vi "MAIN_UI.vi"() -> ()   [LabVIEW 2019]
uses:
  SV_Wrap/shared variable info.ctl
  SV_Wrap/SharedVariableWrapper.lvclass
  Logger_class/Current Alarms.ctl
  Logger_class/EventData.ctl
  TypeDef/AlarmType.ctl
  SV_Wrap/SharedVariableWrapper.lvclass/SharedVariableWrapper.ctl
  TypeDef/error.ctl
  GUI_class/GUI.lvclass/GUI.ctl
  MessageAMC_class/MessageAMC.lvclass
  C:/Users/ANENKOV_V1/Desktop/SRC_H400/src/MessageInterface_class/MessageInterface.lvclass
  ConfigJSON_class/ConfigJSON.lvclass
  TypeDef/Windows.ctl
  GUI Sensor Lib/GUI Sensor Lib.lvclass
  C:/Users/ANENKOV_V1/Desktop/SRC_H400/src/GUI_class/GUI.lvclass
  GUI Alarm Setting/GUI Alarm Setting.lvclass
  GUI Data Viewer_class/GUI Data Viewer.lvclass
  GUI Test Channels_class/GUI Test Channels.lvclass
  GUI Setting_class/GUI Setting.lvclass
  GUI Test HIPRESS_class/GUI Test HIPRESS.lvclass
  GUI NV class/GUI NV.lvclass
  GUI Work Windows_class/GUI Work Windows.lvclass
  PumpMotorGroup_class/GUI PumpMotorGroup.lvclass
  ConfigJSON_class/ConfigJSON.lvclass/ConfigJSON.ctl
  28b6755c-365d-47ee-a391-b63f47e4b467.vi
  4313fddc-c2f7-4c5c-84fc-ac29d5ff3ebf.vi
  d1d2263f-3a8b-4136-8dd0-7d9082776734.vi
  28b6755c-365d-47ee-a391-b63f47e4b467.vi/59a5e995-9048-4616-a220-4159bcf9e391.vi
  SV_Wrap/Write Var Info.vi
  SV_Wrap/Read Var Info.vi
  4313fddc-c2f7-4c5c-84fc-ac29d5ff3ebf.vi/c3b15906-7c69-4354-9ca0-0932e3ff86b4.vi
  GUI_class/Set Win State.vi
  GUI_class/protected/GetSheredData.vi
  SV_Wrap/Read connection str.vi
  <userlib>/_OpenG.lib/time/time.llb/Tick Count (ms)__ogtk.vi
  <vilib>/Platform/browser.llb/Open URL in Default Browser (string).vi
  GUI_class/GUI.lvclass
  <vilib>/NI/AMC/AMC.lvlib
  MessageInterface_class/MessageInterface.lvclass
panel:
  in  "grafana":bool
  out "База данных":bool
  out "Контролер":bool
  in  "Clear error":bool
  in  "Boolean":bool
  out "SVW":refnum<class "SharedVariableWrapper.lvclass">
  in  "Log Out":bool
  in  "Log In":bool
  out "Multicolumn Listbox":i32(listbox)=-1
  out "map":map{string, T1}(c390)
  in  "GUI PMG":bool
  in  "NV2":bool
  in  "NV1":bool
  in  "HI press":bool
  in  "Channel Testing":bool
  in  "Data":bool
  in  "Start Button":bool
  in  "Settings Channels":bool
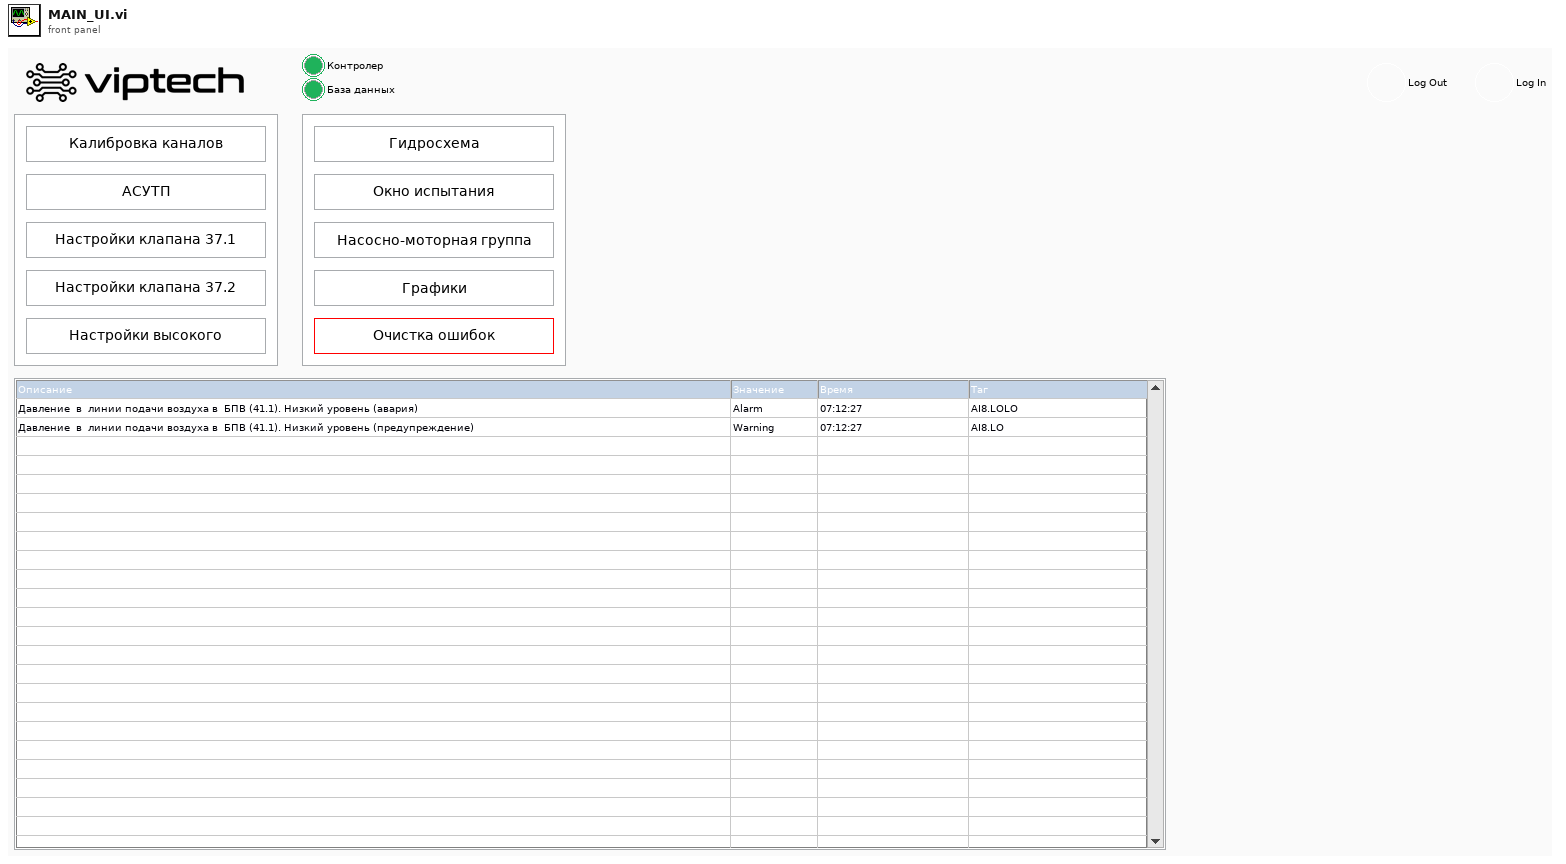
[diagram p1: front panel]
types:
  T1 = typedef "SharedVariableWrapper.lvclass/shared variable info.ctl" = cluster{"shared variable":refnum<k21>, "connected":bool, "Value":variant, "UpdateTime":timestamp}
  T2 = typedef "Current Alarms.ctl" = cluster{"alarms":T3[]}
  T3 = typedef "EventData.ctl" = cluster{"obj_tag":string, "event_tag":string, "Description":string, "ALARM TYPE":T4, "Value DBL":dbl, "Value INT":i32, "Value STR":string, "Time Stamp":timestamp}
  T4 = typedef "AlarmType.ctl" = enum16{"Normal", "Warning", "Alarm"}
  T5 = typedef "error.ctl" = errorcluster
  T6 = enum32{"Invalid", "Standard", "Closed", "Hidden", "Minimized", "Maximized"}
  T7 = enum32{"invalid app kind", "Development System", "Run Time System", "Student Edition", "Embedded LabVIEW", "Evaluation", "Custom"}
  T8 = typedef "Windows.ctl" = cluster{"GUI Sensor Lib":refnum<class "GUI Sensor Lib.lvclass">, "GUI Alarm Setting":refnum<class "GUI Alarm Setting.lvclass">, "GUI Data Viewer":refnum<class "GUI Data Viewer.lvclass">, "GUI Test Channels":refnum<class "GUI Test Channels.lvclass">, "GUI Setting":refnum<class "GUI Setting.lvclass">, "GUI Test HIPRESS":refnum<class "GUI Test HIPRESS.lvclass">, "GUI NV 1":refnum<class "GUI NV.lvclass">, "GUI NV 2":refnum<class "GUI NV.lvclass">, "GUI Work Windows":refnum<class "GUI Work Windows.lvclass">, "GUI PMG 2":refnum<class "GUI PumpMotorGroup.lvclass">}
  T9 = typedef "SharedVariableWrapper.lvclass/Config.ctl" = cluster{"connection str":string, "timeout":dbl, "ip":string}
  T10 = cluster{"Core":cluster{"Current VI Reference":refnum<vi>, "Close Panel on Exit?":bool}, "JSON":refnum<class "ConfigJSON.lvclass">, "SVW":refnum<class "SharedVariableWrapper.lvclass">, "amc":refnum<class "MessageAMC.lvclass">, "Windows":T8}
  T11 = cluster{"Current VI Reference":refnum<vi>, "Close Panel on Exit?":bool}
  T12 = typedef "GUI Paths.ctl" = cluster{"Dir Data":path, "Dir Setting":path, "SensorLib":path, "Dir Scripts":path}
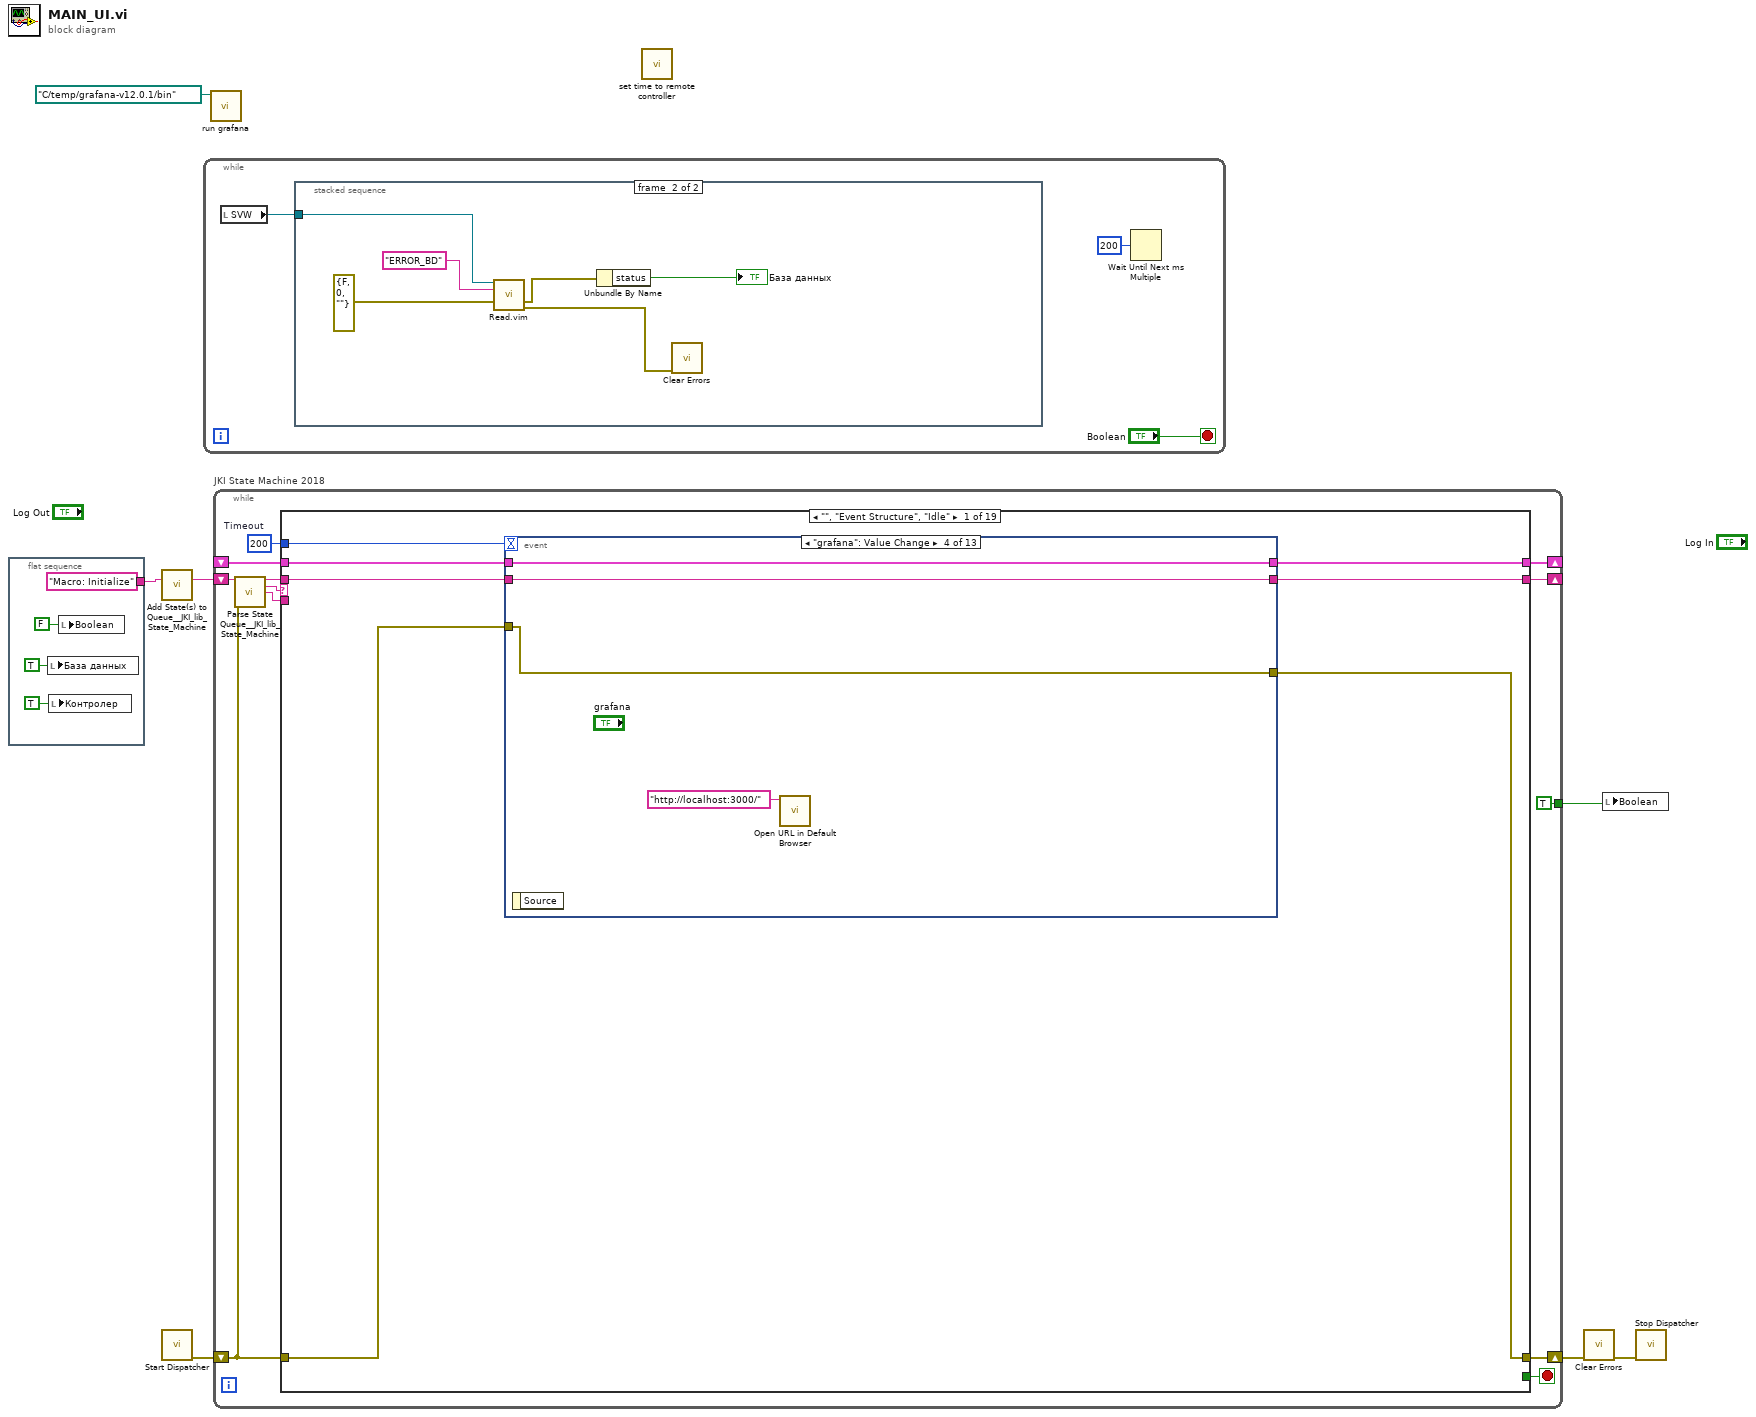
[diagram p0: block diagram]
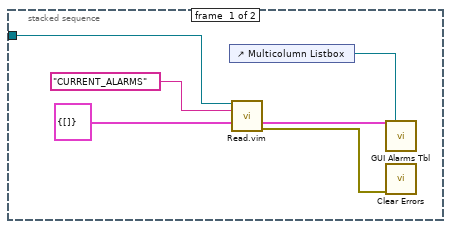
[diagram p2: hidden frame]
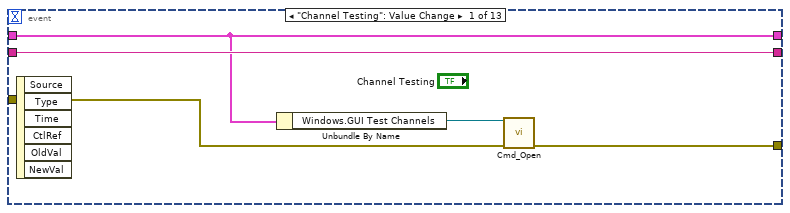
[diagram p3: hidden frame]
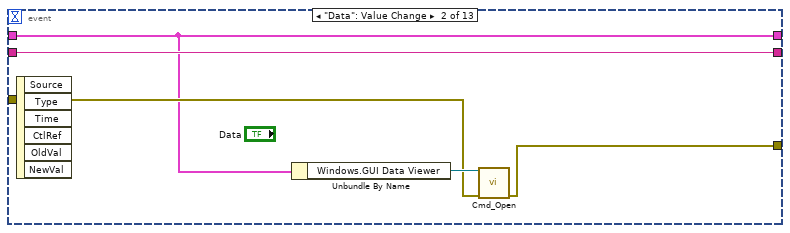
[diagram p4: hidden frame]
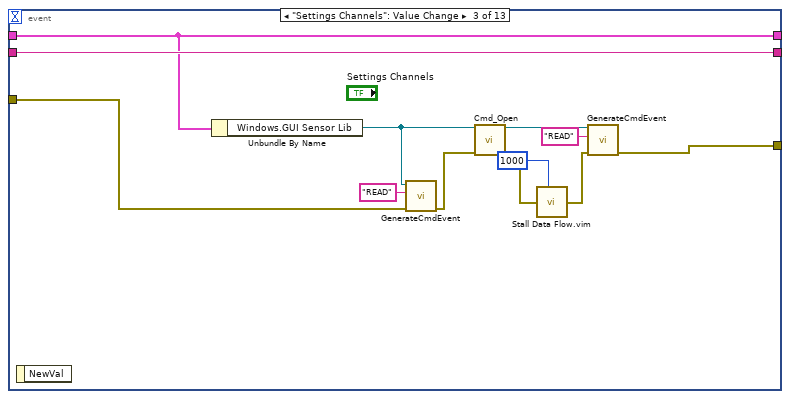
[diagram p5: hidden frame]
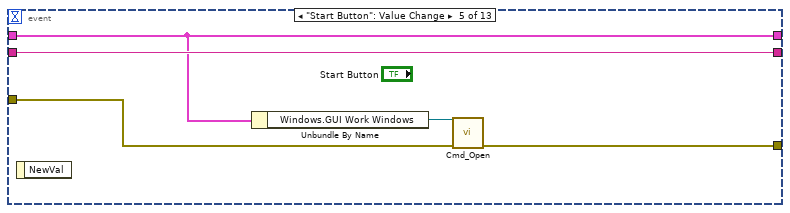
[diagram p6: hidden frame]
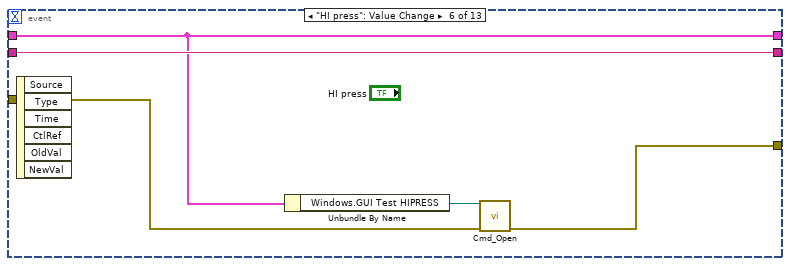
[diagram p7: hidden frame]
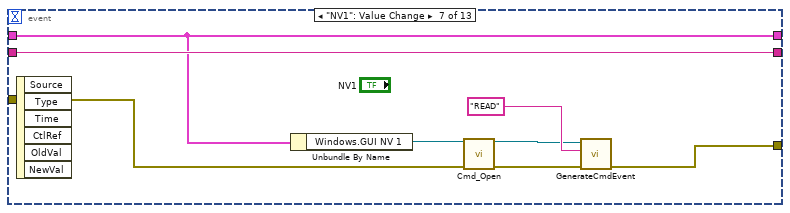
[diagram p8: hidden frame]
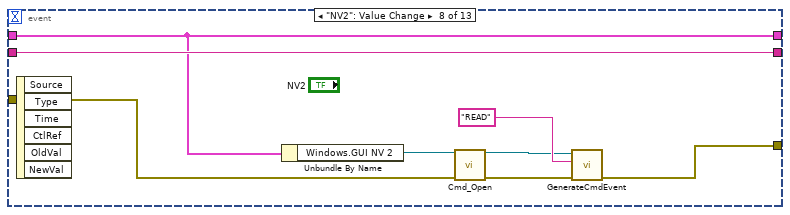
[diagram p9: hidden frame]
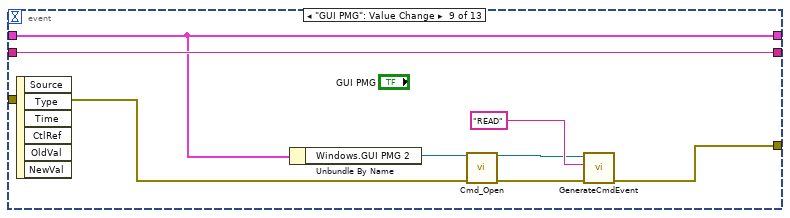
[diagram p10: hidden frame]
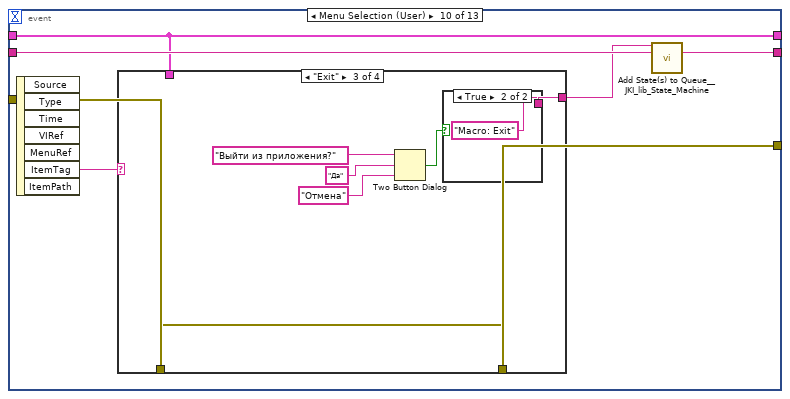
[diagram p11: hidden frame]
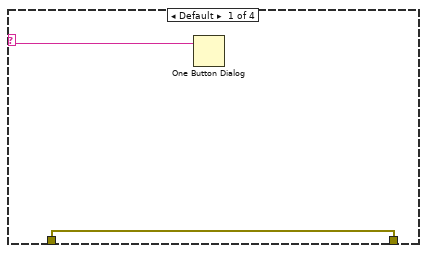
[diagram p12: hidden frame]
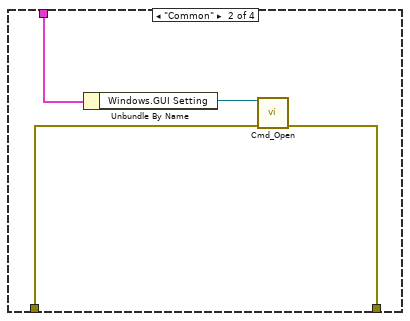
[diagram p13: hidden frame]
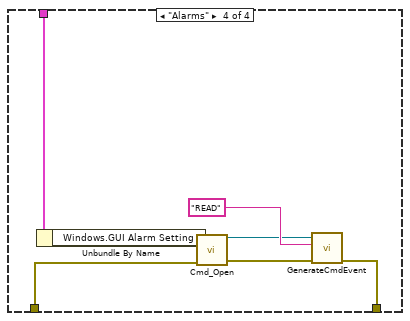
[diagram p15: hidden frame]
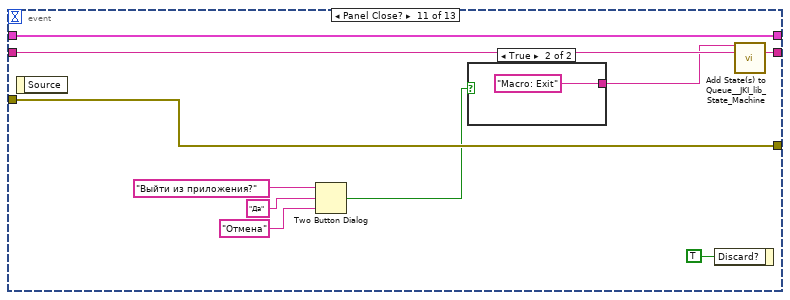
[diagram p16: hidden frame]
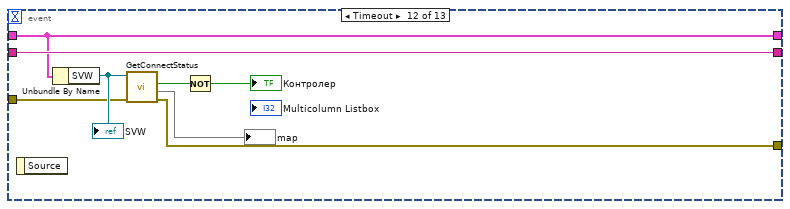
[diagram p18: hidden frame]
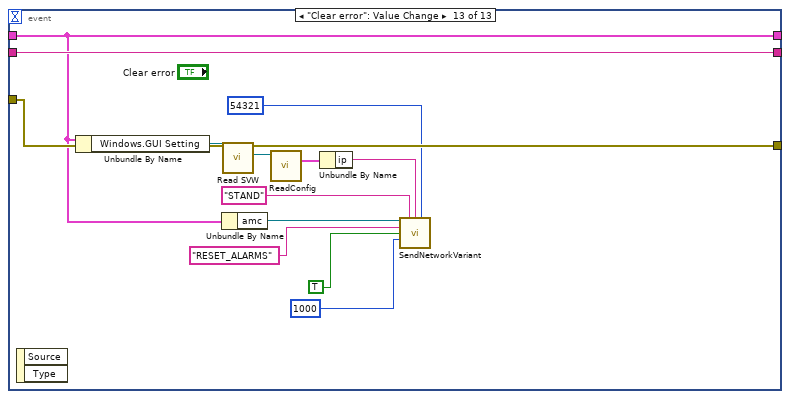
[diagram p19: hidden frame]
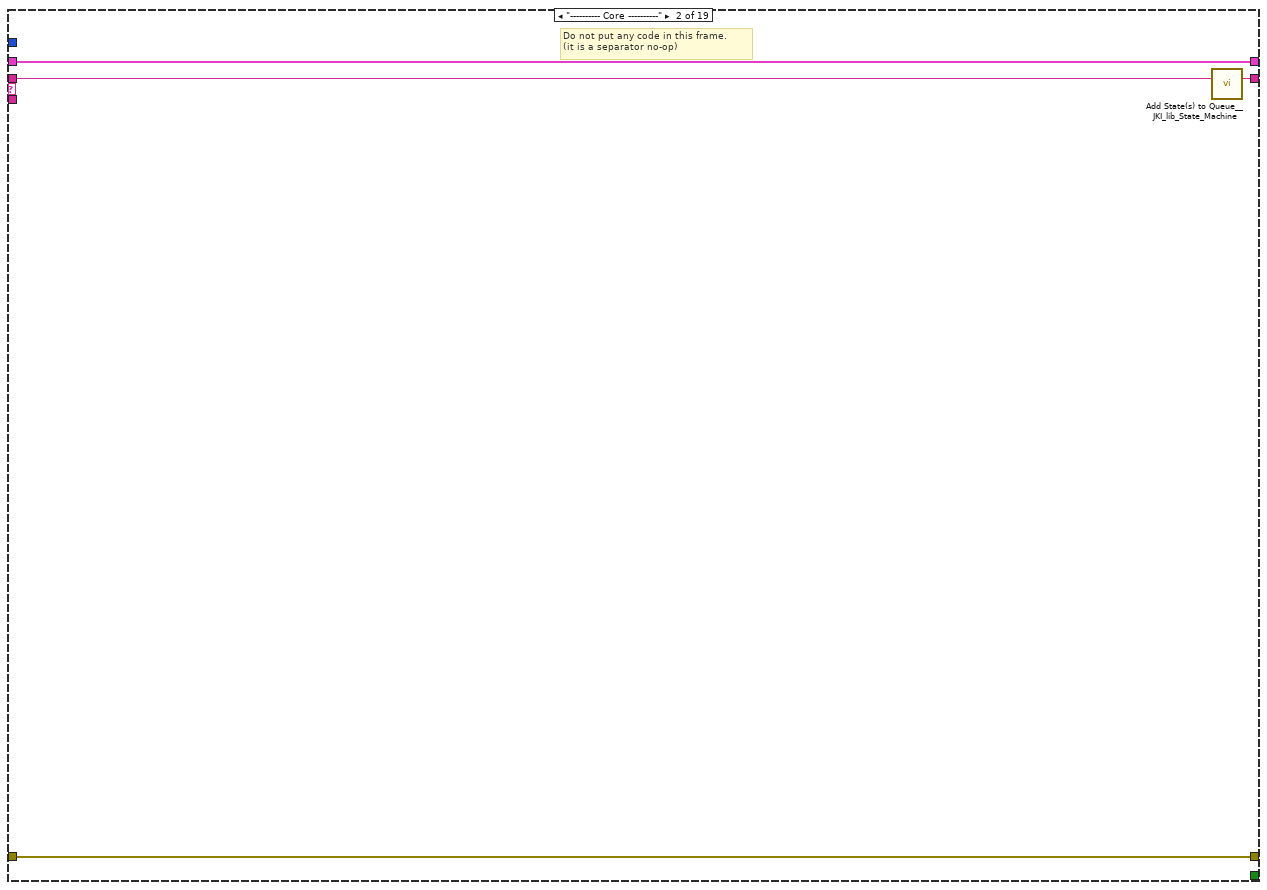
[diagram p20: hidden frame]
diagram:
  n1 = flat-sequence {
    tunnel: ["Macro: Initialize"] -> w2
    frame #0 {
      n2 = local write "База данных"(TRUE ("База данных")) -> ()
      n3 = local write "Контролер"(TRUE ("Контролер")) -> ()
      n4 = local write "Boolean"(FALSE ("Boolean")) -> ()
    }
  }
  n5 = call <vilib>:"Add State(s) to Queue__JKI_lib_State_Machine.vi"("State(s) in (\"\")"=w2) -> ("States Out"=w7:string)  [unwired: 14 in]
  n6 = call <vilib>:"Start Dispatcher.vi"() -> ("error out"=w6:errorcluster)  [unwired: 13 in, 2 out]
  n7 = while {
    stop <- "Boolean" stop-if-true
    n8 = local read "SVW"() -> (w14:refnum<class "SharedVariableWrapper.lvclass">)
    n9 = stacked-sequence {
      tunnel: w14 -> [w16 w25]
      frame #0 {
        n10 = control-ref of="Multicolumn Listbox"() -> (w20:refnum<vi>)
        n11 = call "Read.vim"("SharedVariableWrapper in"=w16, "name"="CURRENT_ALARMS", "DataType"=T2 {"alarms"=[]} ("data out")) -> ("data out"=w19:T2, "error out"=w18:errorcluster)  [unwired: 6 in, 5 out]
        n12 = call "GUI Alarms Tbl.vi"("data in"=w19, "Multicolumn Listbox ref"=w20) -> ()  [unwired: 12 in, 2 out]
        n13 = call <vilib>:"Clear Errors.vi"("error in (no error)"=w18) -> ()  [unwired: 5 in, 2 out]
      }
      frame #1 {
        n14 = call "Read.vim"("SharedVariableWrapper in"=w25, "name"="ERROR_BD", "DataType"=T5 {"status"=FALSE, "code"=0, "source"=""} ("error")) -> ("data out"=w22:T5, "error out"=w24:errorcluster)  [unwired: 6 in, 5 out]
        n15 = Unbundle By Name(w22) -> ("status"=→"База данных":bool)
        n16 = call <vilib>:"Clear Errors.vi"("error in (no error)"=w24) -> ()  [unwired: 5 in, 2 out]
      }
    }
    n17 = Wait Until Next ms Multiple(millisecond multiple=u32 200) -> ()  [unwired: 1 out]
  }
  n18 = call "run grafana.vi"("working directory"=path "C:/temp/grafana-v12.0.1/bin") -> ()  [unwired: 11 in]
  n19 = while "JKI State Machine 2018" {
    shift-right: [w31] -> _
    shift-left: _ -> [w30]
    shift-right: [w34] -> w5
    shift-left: w6 -> [w28]
    shift-right: [w33] -> _
    shift-left: w7 -> [w35]
    tunnel: [TRUE ("Boolean")] -> w3
    stop <- w32 stop-if-true
    w29 = 200  # Timeout
    n20 = call <vilib>:"Parse State Queue__JKI_lib_State_Machine.vi"("State Queue"=w35, "Error In (no error)"=w28) -> ("Remaining States"=w37:string, "Current State"=w38:string, "Arguments"=w36:string)  [unwired: 11 in]
    n21 = case shown="\"\", \"Event Structure\", \"Idle\"" w38 {
      selector: w38 -> [_ _ w169 _ _ _ _ _ _ _ _ _ _ _ _ _ _ _ _]
      tunnel: w37 -> [w45 w168 w173 w192 w198 w203 w207 w225 w231 w235 w239 w245 w256 w325 w330 w341 w345 w350 w361]
      tunnel: w36 -> [_ _ _ _ _ _ _ _ _ _ _ w240 w250 _ _ _ _ _ _]
      tunnel: w30 -> [w43 w165 w171 w185 w195 w201 w204 _ w226 w232 w237 w243 w252 w322 w327 w338 w342 w348 w358]
      tunnel: [w42 w166 w175 w189 errorcluster {"status"=FALSE, "code"=0, "source"=""} ("error out") w200 w205 w210 w227 w233 w236 w241 w253 w323 w328 w339 w343 w349 w359] -> w34
      tunnel: w28 -> [w41 w166 w174 w189 w194 w200 w205 w220 w228 w233 w236 w242 w254 w323 w328 w339 w343 w347 w360]
      tunnel: [w44 w167 w172 w191 w197 w202 w206 w225 w230 w234 w238 w244 w255 w324 w329 w340 w344 w350 w361] -> w33
      tunnel: [_ _ _ _ _ TRUE _ _ _ _ _ _ _ _ _ _ _ _ _] -> w32
      tunnel: [w40 w165 w171 w190 w195 w201 w204 w224 w226 w232 w237 w243 w252 w322 w327 w338 w342 w346 w358] -> w31
      tunnel: w29 -> [w39 _ _ _ _ _ _ _ _ _ _ _ _ _ _ _ _ _ _]
      frame "", "Event Structure", "Idle" {
        n22 = event shown="[3] \"grafana\": Value Change" {
          selector: _ -> [_ _ _ _ _ _ _ _ _ _ _ _ _]
          dyn-events: _ -> [_ _ _ _ _ _ _ _ _ _ _ _ _]
          timeout: w39 -> [_ _ _ _ _ _ _ _ _ _ _ _ _]
          tunnel: w45 -> [w50 w55 w67 w71 w76 w81 w89 w97 w105 w110 w142 w151 w164]
          tunnel: [w50 w55 w67 w71 w76 w81 w89 w97 w105 w111 w141 w151 w164] -> w44
          tunnel: w43 -> [w47 w51 w66 w69 w75 w79 w87 w95 w103 w108 w139 w150 w153]
          tunnel: [w46 w52 w65 w70 w73 w77 w85 w93 w101 w106 w140 w149 w163] -> w42
          tunnel: w41 -> [w48 w53 w60 w70 w74 w78 w86 w94 w102 w107 w140 w147 w163]
          tunnel: [w47 w51 w66 w69 w75 w79 w87 w95 w103 w108 w139 w150 w153] -> w40
          event "Channel Testing": Value Change {
            n23 = event-data() -> ()  [unwired: 1 in, 6 out]
            n24 = Unbundle By Name(w47) -> ("Windows.GUI Test Channels"=w49:refnum<class "GUI Test Channels.lvclass">)
            n25 = call "Cmd_Open.vi"("reference in"=w49, "error in (no error)"=w48) -> ("error out"=w46:errorcluster)  [unwired: 12 in, 1 out]
          }
          event "Data": Value Change {
            n26 = event-data() -> ()  [unwired: 1 in, 6 out]
            n27 = Unbundle By Name(w51) -> ("Windows.GUI Data Viewer"=w54:refnum<class "GUI Data Viewer.lvclass">)
            n28 = call "Cmd_Open.vi"("reference in"=w54, "error in (no error)"=w53) -> ("error out"=w52:errorcluster)  [unwired: 12 in, 1 out]
          }
          event "Settings Channels": Value Change {
            n29 = event-data() -> ()  [unwired: 1 in, 1 out]
            n30 = Unbundle By Name(w66) -> ("Windows.GUI Sensor Lib"=w61:refnum<class "GUI Sensor Lib.lvclass">)
            n31 = call "GenerateCmdEvent.vi"("error in (no error)"=w60, "CMD"="READ", "GUI in"=w61) -> ("error out"=w59:errorcluster)  [unwired: 7 in, 1 out]
            n32 = call "Cmd_Open.vi"("reference in"=w61, "error in (no error)"=w59) -> ("reference out"=w64:refnum<class "GUI Sensor Lib.lvclass">, "error out"=w58:errorcluster)  [unwired: 12 in]
            n33 = call "Stall Data Flow.vim"("value in"=w58, "milliseconds to wait"=u32 1000) -> ("value out"=w57:errorcluster)  [unwired: 1 out]
            n34 = call "GenerateCmdEvent.vi"("error in (no error)"=w57, "CMD"="READ", "GUI in"=w64) -> ("error out"=w65:errorcluster)  [unwired: 7 in, 1 out]
          }
          event "grafana": Value Change {
            n35 = event-data() -> ()  [unwired: 1 in, 1 out]
            n36 = call-poly <vilib>:"Open URL in Default Browser.vi"("URL"="http://localhost:3000/") -> ()  [unwired: 5 in, 2 out]
          }
          event "Start Button": Value Change {
            n37 = event-data() -> ()  [unwired: 1 in, 1 out]
            n38 = Unbundle By Name(w75) -> ("Windows.GUI Work Windows"=w72:refnum<class "GUI Work Windows.lvclass">)
            n39 = call "Cmd_Open.vi"("reference in"=w72, "error in (no error)"=w74) -> ("error out"=w73:errorcluster)  [unwired: 12 in, 1 out]
          }
          event "HI press": Value Change {
            n40 = event-data() -> ()  [unwired: 1 in, 6 out]
            n41 = Unbundle By Name(w79) -> ("Windows.GUI Test HIPRESS"=w80:refnum<class "GUI Test HIPRESS.lvclass">)
            n42 = call "Cmd_Open.vi"("reference in"=w80, "error in (no error)"=w78) -> ("error out"=w77:errorcluster)  [unwired: 12 in, 1 out]
          }
          event "NV1": Value Change {
            n43 = event-data() -> ()  [unwired: 1 in, 6 out]
            n44 = Unbundle By Name(w87) -> ("Windows.GUI NV 1"=w88:refnum<class "GUI NV.lvclass">)
            n45 = call "Cmd_Open.vi"("reference in"=w88, "error in (no error)"=w86) -> ("reference out"=w82:refnum<class "GUI NV.lvclass">, "error out"=w83:errorcluster)  [unwired: 12 in]
            n46 = call "GenerateCmdEvent.vi"("error in (no error)"=w83, "CMD"="READ", "GUI in"=w82) -> ("error out"=w85:errorcluster)  [unwired: 7 in, 1 out]
          }
          event "NV2": Value Change {
            n47 = event-data() -> ()  [unwired: 1 in, 6 out]
            n48 = Unbundle By Name(w95) -> ("Windows.GUI NV 2"=w96:refnum<class "GUI NV.lvclass">)
            n49 = call "Cmd_Open.vi"("reference in"=w96, "error in (no error)"=w94) -> ("reference out"=w90:refnum<class "GUI NV.lvclass">, "error out"=w91:errorcluster)  [unwired: 12 in]
            n50 = call "GenerateCmdEvent.vi"("error in (no error)"=w91, "CMD"="READ", "GUI in"=w90) -> ("error out"=w93:errorcluster)  [unwired: 7 in, 1 out]
          }
          event "GUI PMG": Value Change {
            n51 = event-data() -> ()  [unwired: 1 in, 6 out]
            n52 = Unbundle By Name(w103) -> ("Windows.GUI PMG 2"=w104:refnum<class "GUI PumpMotorGroup.lvclass">)
            n53 = call "Cmd_Open.vi"("reference in"=w104, "error in (no error)"=w102) -> ("reference out"=w98:refnum<class "GUI PumpMotorGroup.lvclass">, "error out"=w99:errorcluster)  [unwired: 12 in]
            n54 = call "GenerateCmdEvent.vi"("error in (no error)"=w99, "CMD"="READ", "GUI in"=w98) -> ("error out"=w101:errorcluster)  [unwired: 7 in, 1 out]
          }
          event Menu Selection (User) {
            n55 = event-data() -> ("ItemTag"=w112:string)  [unwired: 1 in, 6 out]
            n56 = case shown="\"Exit\"" w112 {
              selector: w112 -> [w113 _ _ _]
              tunnel: [_ _ w124 _] -> w109
              tunnel: w108 -> [_ w117 _ w130]
              tunnel: w107 -> [w114 w116 w123 w131]
              tunnel: [w114 w115 w123 w126] -> w106
              frame Default {
                n57 = One Button Dialog(message=w113) -> ()  [unwired: 1 in, 1 out]
              }
              frame "Common" {
                n58 = Unbundle By Name(w117) -> ("Windows.GUI Setting"=w118:refnum<class "GUI Setting.lvclass">)
                n59 = call "Cmd_Open.vi"("reference in"=w118, "error in (no error)"=w116) -> ("error out"=w115:errorcluster)  [unwired: 12 in, 1 out]
              }
              frame "Exit" {
                n60 = Two Button Dialog(message="Выйти из приложения?", 1:"Отмена" ("F button name (\"Cancel\")"), 2:"Да" ("T button name (\"OK\")")) -> (T button?=w119:bool)
                n61 = case shown="True" w119 {
                  tunnel: [_ "Macro: Exit"] -> w124
                  frame False {
                  }
                  frame True {
                  }
                }
              }
              frame "Alarms" {
                n62 = Unbundle By Name(w130) -> ("Windows.GUI Alarm Setting"=w132:refnum<class "GUI Alarm Setting.lvclass">)
                n63 = call "Cmd_Open.vi"("reference in"=w132, "error in (no error)"=w131) -> ("reference out"=w128:refnum<class "GUI Alarm Setting.lvclass">, "error out"=w127:errorcluster)  [unwired: 12 in]
                n64 = call "GenerateCmdEvent.vi"("error in (no error)"=w127, "CMD"="READ", "GUI in"=w128) -> ("error out"=w126:errorcluster)  [unwired: 7 in, 1 out]
              }
            }
            n65 = call <vilib>:"Add State(s) to Queue__JKI_lib_State_Machine.vi"("State(s) in Front (\"\")"=w109, "State(s) in (\"\")"=w110) -> ("States Out"=w111:string)  [unwired: 13 in]
          }
          event Panel Close? {
            n66 = event-data() -> ()  [unwired: 1 in, 1 out]
            n67 = Two Button Dialog(message="Выйти из приложения?", 1:"Отмена" ("F button name (\"Cancel\")"), 2:"Да" ("T button name (\"OK\")")) -> (T button?=w133:bool)
            n68 = case shown="True" w133 {
              tunnel: [_ "Macro: Exit"] -> w138
              frame False {
              }
              frame True {
              }
            }
            n69 = event-data("Discard?"=TRUE) -> ()  [unwired: 1 in, 1 out]
            n70 = call <vilib>:"Add State(s) to Queue__JKI_lib_State_Machine.vi"("State(s) in Front (\"\")"=w138, "State(s) in (\"\")"=w142) -> ("States Out"=w141:string)  [unwired: 13 in]
          }
          event Timeout {
            n71 = event-data() -> ()  [unwired: 1 in, 1 out]
            n72 = Unbundle By Name(w150) -> ("SVW"=w148:refnum<class "SharedVariableWrapper.lvclass">)
            "SVW" <- w148
            n73 = call "GetConnectStatus.vi"("error in (no error)"=w147, "SharedVariableWrapper in"=w148) -> ("error out"=w149:errorcluster, "map"=→"map":map{string, T1}, "Connected?"=w145:bool)  [unwired: 7 in]
            n74 = Not(x=w145) -> (.not. x?=→"Контролер":bool)
          }
          event "Clear error": Value Change {
            n75 = event-data() -> ()  [unwired: 1 in, 2 out]
            n76 = Unbundle By Name(w153) -> ("Windows.GUI Setting"=w152:refnum<class "GUI Setting.lvclass">)
            n77 = Unbundle By Name(w153) -> ("amc"=w159:refnum<class "MessageAMC.lvclass">)
            n78 = call "Read SVW.vi"("GUI in"=w152) -> ("SharedVariableWrapper.lvclass"=w160:refnum<class "SharedVariableWrapper.lvclass">)  [unwired: 10 in]
            n79 = call "ReadConfig.vi"("SharedVariableWrapper in"=w160) -> ("config"=w161:T9)  [unwired: 12 in, 2 out]
            n80 = Unbundle By Name(w161) -> ("ip"=w162:string)
            n81 = call "SendNetworkVariant.vi"("reference in"=w159, "receiver process"="STAND", "receiver host"=w162, "receiver port (0)"=u16 54321, "name"="RESET_ALARMS", "data"=TRUE, "timeout (25000 ms)"=1000) -> ()  [unwired: 6 in, 3 out]
          }
        }
      }
      frame "---------- Core ----------" {
        # "Do not put any code in this frame.\n(it is a separator no-op)"
        n82 = call <vilib>:"Add State(s) to Queue__JKI_lib_State_Machine.vi"("State(s) in (\"\")"=w168) -> ("States Out"=w167:string)  [unwired: 14 in]
      }
      frame Default {
        w178 = 42 items=["No error", "Argument error", "Memory is full", "Out of zone", "End of file", "File already open", "Generic file I/O error", "File not found", "File permission error", "Disk is full", "Duplicate path", "Too many files open", "System feature not enabled", "Resource file not found", "Cannot add resource", "Resource not found", "Image not found", "Image memory error", "Pen does not exist", "Config type invalid", "Config token not found", "Config parse error", "Config memory error", "Bad external code format", "Bad external code offset", "External code not present", "Null window", "Destroy window error", "Null menu", "Print aborted", "Bad print record", "Print driver error", "Windows error during printing", "Memory error during printing", "Print dialog error", "Generic print error", "Invalid device refnum", "Device not found", "Device parameter error", "Device unit error", "Cannot open device", "Device call aborted", "Generic error", "Cancelled by user", "Object ID too low", "Object ID too high", "Object not in heap", "Unknown heap", "Unknown object (invalid DefProc)", "Unknown object (DefProc not in table)", "Message out of range", "Invalid (null) method", "Unknown message", "Manager call not supported", "Bad address", "Network operation in progress", "Network operation timed out", "Connection is busy", "Network attribute not supported", "Network error", "Address in use", "System out of memory", "Connection aborted", "Connection refused", "Not connected", "Already connected", "Connection closed", "Initialization error (interapplication manager)", "Bad occurrence", "Wait on unbound occurrence handler", "Occurrence queue overflow", "Datalog type conflict", "Unused", "Unrecognized type (interapplication manager)", "Memory corrupt", "Failed to make temporary DLL", "Old CIN version", "Drag socket not found", "Failed to load drop-object", "Failed to register OLE object", "Failed to release OLE object", "Format specifier type mismatch", "Unknown format specifier", "Too few format specifiers", "Too many format specifiers", "Scan failed", "Newer CIN version", "Error converting to variant", "Runtime menu error", "Password tampered", "Variant attribute not found", "Incompatible variant data type", "Event data is not available", "Event Store is not present", "Occurrence is not found", "Event Queue is not created", "Event info is not available", "Refnum passed is NULL", "Error retrieving Class GUID", "Error retrieving CoClass GUID", "Error retrieving TypeLib GUID.", "Bad built application magic bytes.", "Specific driver is different from the specific driver associated with the Logical Name.", "There is no session opened to the class driver.", "Max Error", "MAX - Error with config objects", "MAX - Error loading configuration", "MAX - Group not supported"]
        # "Current State"
        # "Do not delete, rename, or modify this frame.\n(this is used to capture unhandled states and typos)"
        # "Handle mistyped state name (developer tool)"
        n83 = Format Into String(format string="Software Exception: Unhandled State \"%s\"." ("message"), error in=w174, w169) -> (resulting string=w177:string, error out=w176:errorcluster)  [unwired: 1 in]
        n84 = call <vilib>:"Error Cluster From Error Code.vi"("show call chain? (False)"=TRUE, "error in (no error)"=w176, "error message (\"\")"=w177, "error code (0)"=w178) -> ("error out"=w175:errorcluster)  [unwired: 5 in]
        n85 = call <vilib>:"Add State(s) to Queue__JKI_lib_State_Machine.vi"("State(s) in (\"\")"=w173) -> ("States Out"=w172:string)  [unwired: 14 in]
      }
      frame "Initialize Core Data" {
        # "Do not delete, rename, or modify this frame.\n(this is used to determine panel behavior on exit)"
        # "originally closed?"
        # "exe?"
        # "If panel starts closed or is an EXE, then close it when we exit"
        n86 = property class="VI"() -> ("FP.State"=w182:T6)  [unwired: 2 in, 2 out]
        n87 = property class="App"() -> ("App.Kind"=w188:T7)  [unwired: 2 in, 2 out]
        n88 = control-ref of="Current VI Reference"() -> (w183:refnum<vi>)
        n89 = Equal?(x=w182, y=T6."Closed" ("Front Panel Window:State")) -> (x = y?=w180:bool)
        n90 = Equal?(x=w188, y=T7."Run Time System" ("Application:Kind")) -> (x = y?=w186:bool)
        n91 = Or(x=w180, y=w186) -> (x .or. y?=w184:bool)
        n92 = Bundle By Name(cluster=w185, "Core.Current VI Reference"=w183, "Core.Close Panel on Exit?"=w184) -> (w190:T10)
        n93 = call <vilib>:"Add State(s) to Queue__JKI_lib_State_Machine.vi"("State(s) in (\"\")"=w192) -> ("States Out"=w191:string)  [unwired: 14 in]
      }
      frame "Error Handler" {
        # "Unhandled Error -- Display it"
        # "Handle any errors here.\nYou can also output any states to clean-up after errors occur"
        # "Clear error"
        n94 = call <vilib>:"General Error Handler.vi"("error in (no error)"=w194) -> ()  [unwired: 10 in, 5 out]
        n95 = call <vilib>:"Add State(s) to Queue__JKI_lib_State_Machine.vi"("State(s) in Front (\"\")"="/* Post Error States", "State(s) in (\"\")"=w198) -> ("States Out"=w197:string)  [unwired: 13 in]
      }
      frame "Exit" {
        # "Do not put any code in this frame.\n(No errors that occur here will be handled.)"
        n96 = call <vilib>:"Add State(s) to Queue__JKI_lib_State_Machine.vi"("State(s) in (\"\")"=w203) -> ("States Out"=w202:string)  [unwired: 14 in]
      }
      frame "---------- Data ----------" {
        # "Do not put any code in this frame.\n(It is a separator no-op. You can make a copy of this frame to create a new Data frame)"
        n97 = call <vilib>:"Add State(s) to Queue__JKI_lib_State_Machine.vi"("State(s) in (\"\")"=w207) -> ("States Out"=w206:string)  [unwired: 14 in]
      }
      frame "Data: Initialize" {
        w223 = T11 {"Current VI Reference"=refnum, "Close Panel on Exit?"=FALSE}  # Core
        n98 = call "GUI Get Paths.vi"("error in (no error)"=w220) -> ("Paths"=w221:T12, "error out"=w215:errorcluster)  [unwired: 13 in]
        n99 = Unbundle By Name(w221) -> ("Dir Setting"=w219:path)
        n100 = call "Init.vi"("host"="192.168.1.10", "lib"="RT_Shared_Variables", "update timeout"=0.0, "error in (no error)"=w215) -> ("SVW"=w211:refnum<class "SharedVariableWrapper.lvclass">, "error out"=w210:errorcluster)  [unwired: 10 in]
        n101 = call "SetDir.vi"("reference in"=refnum<class "ConfigJSON.lvclass"> refnum ("ConfigJSON"), "Config Dir"=w219) -> ("JSON"=w212:refnum<class "ConfigJSON.lvclass">)  [unwired: 13 in]
        n102 = call "MessageAMC_Create.vi"("reference in"=refnum<class "MessageAMC.lvclass"> refnum, "error in (no error)"=w210, "message queue name"="MAIN_UI") -> ("amc"=w209:refnum<class "MessageAMC.lvclass">)  [unwired: 15 in, 1 out]
        n103 = Bundle("Core"=w223, "JSON"=w212, "SVW"=w211, "amc"=w209, "Windows"=T8 {"GUI Sensor Lib"=refnum, "GUI Alarm Setting"=refnum, "GUI Data Viewer"=refnum, "GUI Test Channels"=refnum, "GUI Setting"=refnum, "GUI Test HIPRESS"=refnum, "GUI NV 1"=refnum, "GUI NV 2"=refnum, "GUI Work Windows"=refnum, "GUI PMG 2"=refnum}) -> (w224:T10)  [unwired: 1 in]
      }
      frame "Data: Cleanup" {
        # "Cleanup any data and references, here.\n(this is called automatically, by the Macro: Exit)"
        n104 = Unbundle By Name(w226) -> ("Core.Current VI Reference"=w229:refnum<vi>)
        n105 = Close Reference(reference=w229, error in (no error)=w228) -> (error out=w227:errorcluster)
        n106 = call <vilib>:"Add State(s) to Queue__JKI_lib_State_Machine.vi"("State(s) in (\"\")"=w231) -> ("States Out"=w230:string)  [unwired: 14 in]
      }
      frame "---------- UI ----------" {
        # "Do not put any code in this frame.\n(It is a separator no-op. You can make a copy of this frame to create a new UI frame)"
        n107 = call <vilib>:"Add State(s) to Queue__JKI_lib_State_Machine.vi"("State(s) in (\"\")"=w235) -> ("States Out"=w234:string)  [unwired: 14 in]
      }
      frame "UI: Initialize" {
        n108 = call <vilib>:"Add State(s) to Queue__JKI_lib_State_Machine.vi"("State(s) in (\"\")"=w239) -> ("States Out"=w238:string)  [unwired: 14 in]
      }
      frame "UI: Cursor Set" {
        # "Argument"
        # "Set and Unset Cursor Busy.\n(Usage: \"UI: Cursor Set >> Busy|Idle\")"
        n109 = case shown="\"Idle\", Default" w240 {
          tunnel: w242 -> [w247 w249]
          tunnel: [w246 w248] -> w241
          frame "Idle", Default {
            n110 = call <vilib>:"Unset Busy.vi"("error in (no error)"=w247) -> ("error out"=w246:errorcluster)  [unwired: 10 in]
          }
          frame "Busy" {
            n111 = call <vilib>:"Set Busy.vi"("error in (no error)"=w249) -> ("error out"=w248:errorcluster)  [unwired: 9 in, 1 out]
          }
        }
        n112 = call <vilib>:"Add State(s) to Queue__JKI_lib_State_Machine.vi"("State(s) in (\"\")"=w245) -> ("States Out"=w244:string)  [unwired: 14 in]
      }
      frame "UI: Front Panel State" {
        # "Argument"
        # "Set Front Panel Open or Closed\n(Usage: \"UI: Front Panel State >> Open|Close\")"
        n113 = Unbundle By Name(w252) -> ("Core.Current VI Reference"=w251:refnum<vi>)
        n114 = case shown="\"Minimize\", \"Minimized\"" w250 {
          tunnel: w254 -> [w262 w277 w288 w301 w314]
          tunnel: [w264 w278 w290 w303 w316] -> w253
          tunnel: w251 -> [w263 w275 w289 w302 w315]
          frame "Open", "Standard", Default {
            w257 = T6."Standard" ("State")
            n115 = property class="VI"(reference=w263, error in=w262) -> (reference out=w260:refnum<vi>, error out=w261:errorcluster, "FP.State"=w259:T6)
            n116 = Not Equal?(x=w259, y=w257) -> (x != y?=w258:bool)
            n117 = case shown="True" w258 {
              tunnel: [w268 w270] -> w264
              tunnel: w261 -> [w267 w270]
              tunnel: w260 -> [w266 _]
              tunnel: w257 -> [w265 _]
              frame True {
                n118 = invoke class="VI" method="FP.Open"(reference=w266, error in=w267, "Activate"=TRUE, "State"=w265) -> (error out=w268:errorcluster)  [unwired: 1 in, 4 out]
              }
              frame False {
              }
            }
          }
          frame "Close", "Closed" {
            n119 = property class="VI"(reference=w275, error in=w277) -> (reference out=w274:refnum<vi>, error out=w276:errorcluster, "FP.State"=w272:T6)
            n120 = Not Equal?(x=w272, y=T6."Closed" ("Front Panel Window:State")) -> (x != y?=w271:bool)
            n121 = case shown="True" w271 {
              tunnel: [w279 w282] -> w278
              tunnel: w276 -> [w279 w281]
              tunnel: w274 -> [_ w280]
              frame False {
              }
              frame True {
                n122 = invoke class="VI" method="FP.Close"(reference=w280, error in=w281) -> (error out=w282:errorcluster)  [unwired: 1 in, 2 out]
              }
            }
          }
          frame "Hidden", "Hide" {
            w283 = T6."Hidden" ("State")
            n123 = property class="VI"(reference=w289, error in=w288) -> (reference out=w286:refnum<vi>, error out=w287:errorcluster, "FP.State"=w285:T6)
            n124 = Not Equal?(x=w285, y=w283) -> (x != y?=w284:bool)
            n125 = case shown="True" w284 {
              tunnel: [w294 w295] -> w290
              tunnel: w287 -> [w293 w295]
              tunnel: w286 -> [w292 _]
              tunnel: w283 -> [w291 _]
              frame True {
                n126 = invoke class="VI" method="FP.Open"(reference=w292, error in=w293, "State"=w291) -> (error out=w294:errorcluster)  [unwired: 2 in, 4 out]
              }
              frame False {
              }
            }
          }
          frame "Minimize", "Minimized" {
            w296 = T6."Minimized" ("State")
            n127 = property class="VI"(reference=w302, error in=w301) -> (reference out=w299:refnum<vi>, error out=w300:errorcluster, "FP.State"=w298:T6)
            n128 = Not Equal?(x=w298, y=w296) -> (x != y?=w297:bool)
            n129 = case shown="True" w297 {
              tunnel: [w307 w308] -> w303
              tunnel: w300 -> [w306 w308]
              tunnel: w299 -> [w305 _]
              tunnel: w296 -> [w304 _]
              frame True {
                n130 = invoke class="VI" method="FP.Open"(reference=w305, error in=w306, "State"=w304) -> (error out=w307:errorcluster)  [unwired: 2 in, 4 out]
              }
              frame False {
              }
            }
          }
          frame "Maximize", "Maximized" {
            w309 = T6."Maximized" ("State")
            n131 = property class="VI"(reference=w315, error in=w314) -> (reference out=w312:refnum<vi>, error out=w313:errorcluster, "FP.State"=w311:T6)
            n132 = Not Equal?(x=w311, y=w309) -> (x != y?=w310:bool)
            n133 = case shown="True" w310 {
              tunnel: [w320 w321] -> w316
              tunnel: w313 -> [w319 w321]
              tunnel: w312 -> [w318 _]
              tunnel: w309 -> [w317 _]
              frame True {
                n134 = invoke class="VI" method="FP.Open"(reference=w318, error in=w319, "State"=w317) -> (error out=w320:errorcluster)  [unwired: 2 in, 4 out]
              }
              frame False {
              }
            }
          }
        }
        n135 = call <vilib>:"Add State(s) to Queue__JKI_lib_State_Machine.vi"("State(s) in (\"\")"=w256) -> ("States Out"=w255:string)  [unwired: 14 in]
      }
      frame "---------- Macro ----------" {
        # "Do not put any code in this frame.\n(It is a separator no-op. You can make a copy of this frame to create a new Macro frame)"
        n136 = call <vilib>:"Add State(s) to Queue__JKI_lib_State_Machine.vi"("State(s) in (\"\")"=w325) -> ("States Out"=w324:string)  [unwired: 14 in]
      }
      frame "Macro: Initialize" {
        n137 = call <vilib>:"Add State(s) to Queue__JKI_lib_State_Machine.vi"("State(s) in Front (\"\")"="Data: Initialize\nInitialize Core Data\nUI: Initialize\nUI: Front Panel State >> Open\n\nAction: Init GUI", "State(s) in (\"\")"=w330) -> ("States Out"=w329:string)  [unwired: 13 in]
      }
      frame "Macro: Exit" {
        n138 = Unbundle By Name(w338) -> ("Core.Close Panel on Exit?"=w337:bool)
        n139 = Select(t="UI: Front Panel State >> Close", s=w337, f="") -> (s? t:f=w334:string)
        n140 = call <vilib>:"Add State(s) to Queue__JKI_lib_State_Machine.vi"("State(s) in Front (\"\")"="Action: Close GUI\n\n\n", "State(s) in (\"\")"=w334, "State(s) at Back (\"\")"="Data: Cleanup\nExit") -> ("States Out"=w332:string)  [unwired: 12 in]
        n141 = call <vilib>:"Add State(s) to Queue__JKI_lib_State_Machine.vi"("State(s) in Front (\"\")"=w332, "State(s) in (\"\")"=w341) -> ("States Out"=w340:string)  [unwired: 13 in]
      }
      frame "---------- Action ----------" {
        # "Template Separator\n(You can make a copy of, or modify, this frame)"
        n142 = call <vilib>:"Add State(s) to Queue__JKI_lib_State_Machine.vi"("State(s) in (\"\")"=w345) -> ("States Out"=w344:string)  [unwired: 14 in]
      }
      frame "Action: Init GUI" {
        n143 = in-place {
          in-place-border: [w356] -> w349
          in-place-border: w347 -> [w351]
          n144 = in-place-cluster #1(w348) -> ("SVW"=w353:refnum<class "SharedVariableWrapper.lvclass">, "JSON"=w354:refnum<class "ConfigJSON.lvclass">, "Windows"=w355:T8)
          n145 = call "Init GUIs.vi"("Windows in"=w355, "JSON"=w354, "SVW"=w353, "error in"=w351) -> ("Windows out"=w352:T8, "error out"=w356:errorcluster)  [unwired: 10 in]
          n146 = in-place-cluster #1("SVW"=w353, "JSON"=w354, "Windows"=w352) -> (w346:T10)
        }
      }
      frame "Action: Close GUI" {
        n147 = Unbundle By Name(w358) -> ("Windows"=w357:T8)
        n148 = call "Close GUIs.vi"("Windows"=w357, "error in (no error)"=w360) -> ("error out"=w359:errorcluster)  [unwired: 13 in]
      }
    }
  }
  n149 = call "set time to remote controller.vi"() -> ()  [unwired: 12 in]
  n150 = call <vilib>:"Clear Errors.vi"("error in (no error)"=w5) -> ("error out"=w4:errorcluster)  [unwired: 5 in, 1 out]
  n151 = local write "Boolean"(w3) -> ()
  n152 = call <vilib>:"Stop Dispatcher.vi"("error in"=w4) -> ()  [unwired: 14 in, 1 out]
